vi "StreamTransmitAcquisitionChB.vi"() -> ()   [LabVIEW 2012]
uses:
  <resource>/objmgr/ni.dex.rc
panel:
  in  "stop":bool
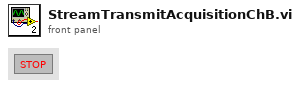
[diagram p1: front panel]
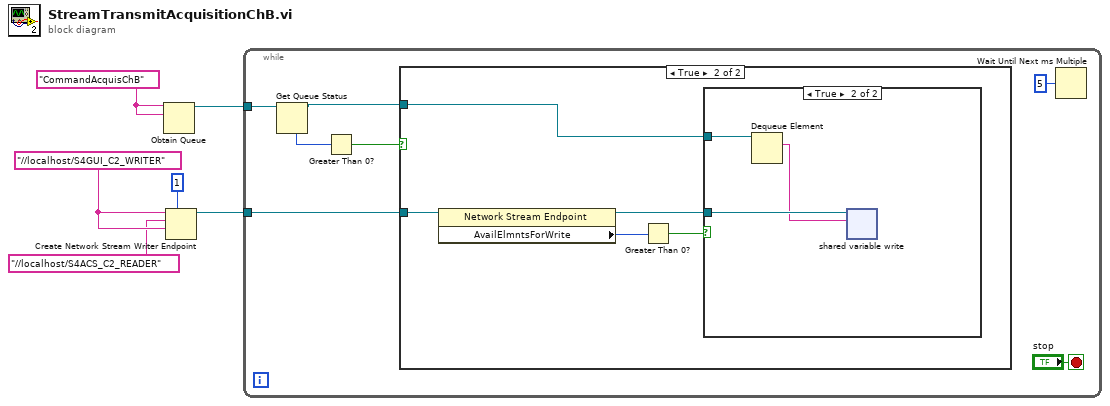
[diagram p0: block diagram]
diagram:
  w3 = "//localhost/S4GUI_C2_WRITER"
  w5 = "CommandAcquisChB"
  n1 = Obtain Queue(name (unnamed)=w5, element data type=w5) -> (queue out=w6:refnum<queue>)  [unwired: 3 in, 2 out]
  n2 = Create Network Stream Writer Endpoint(7:1 ("writer buffer size"), 9:w3, 10:"//localhost/S4ACS_C2_READER", 11:w3) -> (3:w1:refnum<k21>)  [unwired: 3 in, 1 out]
  n3 = while {
    tunnel: w6 -> [w12]
    tunnel: w1 -> [w8]
    stop <- "stop" stop-if-true
    n4 = Get Queue Status(queue=w12) -> (queue out=w9:refnum<queue>, # elements in queue=w11:i32)  [unwired: 2 in, 6 out]
    n5 = Greater Than 0?(x=w11) -> (x > 0?=w10:bool)
    n6 = case shown="True" w10 {
      tunnel: w9 -> [_ w18]
      tunnel: w8 -> [_ w17]
      frame False {
      }
      frame True {
        n7 = property class="Network Stream Endpoint"(reference=w17) -> (reference out=w15:refnum<k21>, "AvailElmntsForWrite"=w16:i32)  [unwired: 1 in, 1 out]
        n8 = Greater Than 0?(x=w16) -> (x > 0?=w14:bool)
        n9 = case shown="True" w14 {
          tunnel: w18 -> [_ w21]
          tunnel: w15 -> [_ w20]
          frame False {
          }
          frame True {
            n10 = Dequeue Element(queue=w21) -> (element=w19:string)  [unwired: 2 in, 3 out]
            n11 = shared-variable-write(w20, w19) -> ()  [unwired: 2 in, 3 out]
          }
        }
      }
    }
    n12 = Wait Until Next ms Multiple(millisecond multiple=u32 5) -> ()  [unwired: 1 out]
  }
